vi "_FPGA Set LCD Msg.vi"(4 "Info":string, 5 "ErrNum":string, 6 "error in":errorcluster, 7 "Line2Msg (same)":T1 items=["Same", "Empty", "VacFail", "Cancel", "CheckGas", "EleFail", "Probe1Fail", "Probe2Fail", "HeaterFail", "DoorOpen", "CheckComm", "PressStart", "CheckSource", "VacWarn", "ForelineHigh", "SourceExhaustLow"], 8 "Line1Msg (same)":T2 items=["Same", "Empty", "Connected", "Starting", "Stopping", "Action", "On", "Service", "Call", "Acquiring", "Source"]) -> (0 "error out":errorcluster)   [LabVIEW 2015]
uses:
  Type/_LCD Line1 Msg.ctl
  Type/_LCD Line2 Msg.ctl
  Type/_RT LED Num.ctl
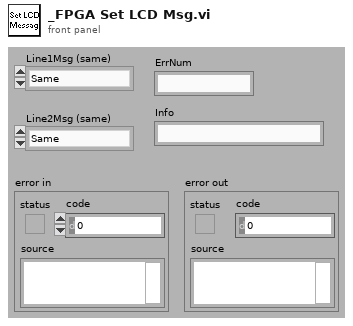
[diagram p1: front panel]
types:
  T1 = typedef "_LCD Line2 Msg.ctl" = u16
  T2 = typedef "_LCD Line1 Msg.ctl" = u16
  T3 = typedef "_RT LED Num.ctl" = enum8{"ReadKey", "ClearKeyBuffer", "ClearLCD", "BacklightOn"}
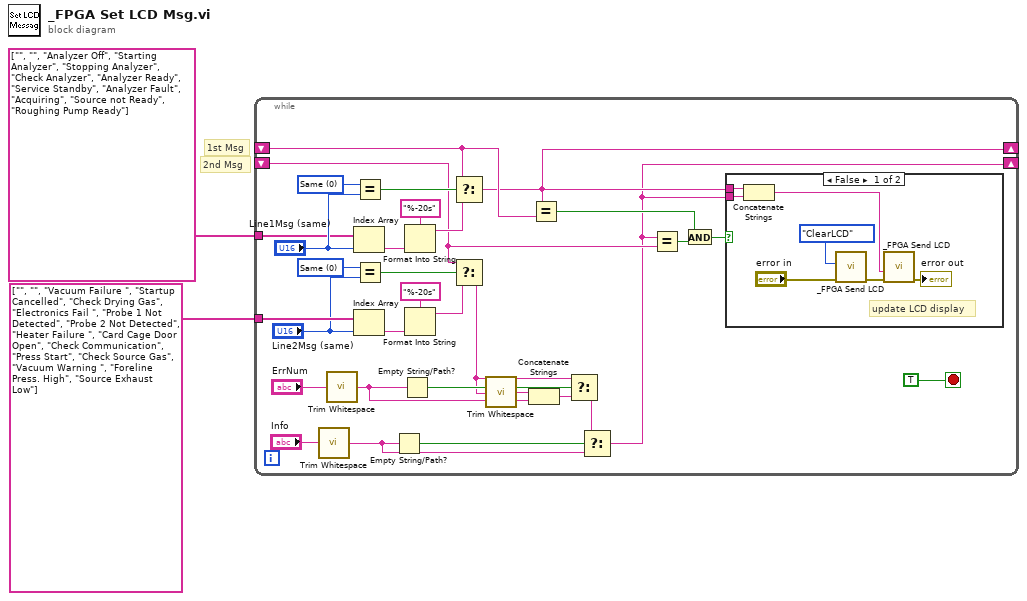
[diagram p0: block diagram]
diagram:
  # "2nd Msg"
  # "1st Msg"
  n1 = while {
    shift-right: [w5] -> _
    shift-left: _ -> [w10]
    shift-right: [w4] -> _
    shift-left: _ -> [w9]
    tunnel: string[] ["", "", "Analyzer Off", "Starting Analyzer", "Stopping Analyzer", "Check Analyzer", "Analyzer Ready", "Service Standby", "Analyzer Fault", "Acquiring", "Source not Ready", "Roughing Pump Ready"] -> [w27]
    tunnel: string[] ["", "", "Vacuum Failure ", "Startup Cancelled", "Check Drying Gas", "Electronics Fail ", "Probe 1 Not Detected", "Probe 2 Not Detected", "Heater Failure ", "Card Cage Door Open", "Check Communication", "Press Start", "Check Source Gas", "Vacuum Warning ", "Foreline Press. High", "Source Exhaust Low"] -> [w22]
    stop <- TRUE stop-if-true
    w20 = T1 0 items=["Same", "Empty", "VacFail", "Cancel", "CheckGas", "EleFail", "Probe1Fail", "Probe2Fail", "HeaterFail", "DoorOpen", "CheckComm", "PressStart", "CheckSource"] ("x")
    w30 = T2 0 items=["Same", "Empty", "Connected", "Starting", "Stopping", "Action", "On", "Service", "Call", "Acquiring", "Source"] ("x")
    n2 = call <vilib>:"Trim Whitespace.vi"("string"="Info") -> ("trimmed string"=w11:string)  [unwired: 1 in]
    n3 = call <vilib>:"Trim Whitespace.vi"("string"="ErrNum") -> ("trimmed string"=w15:string)  [unwired: 1 in]
    n4 = Index Array(array=w27, index="Line1Msg (same)") -> (element=w32:string)
    n5 = Index Array(array=w22, index="Line2Msg (same)") -> (element=w24:string)
    n6 = Equal?(x=w30, y="Line1Msg (same)") -> (x = y?=w29:bool)
    n7 = Equal?(x=w20, y="Line2Msg (same)") -> (x = y?=w25:bool)
    n8 = Empty String/Path?(string/path=w11) -> (empty?=w13:bool)
    n9 = Empty String/Path?(string/path=w15) -> (empty?=w18:bool)
    n10 = Format Into String(format string="%-20s", w32) -> (resulting string=w28:string)  [unwired: 2 in, 1 out]
    n11 = Format Into String(format string="%-20s", w24) -> (resulting string=w26:string)  [unwired: 2 in, 1 out]
    n12 = Select(t=w10, s=w29, f=w28) -> (s? t:f=w5:string)
    n13 = Select(t=w9, s=w25, f=w26) -> (s? t:f=w16:string)
    n14 = call <vilib>:"Trim Whitespace.vi"("string"=w16) -> ("trimmed string"=w3:string)  [unwired: 1 in]
    n15 = Concatenate Strings(w3, w15) -> (w17:string)
    n16 = Equal?(x=w5, y=w10) -> (x = y?=w7:bool)
    n17 = Select(t=w16, s=w18, f=w17) -> (s? t:f=w12:string)
    n18 = Select(t=w12, s=w13, f=w11) -> (s? t:f=w4:string)
    n19 = Equal?(x=w4, y=w9) -> (x = y?=w8:bool)
    n20 = And(x=w7, y=w8) -> (x .and. y?=w6:bool)
    n21 = case shown="False" w6 {
      tunnel: w5 -> [w37 _]
      tunnel: w4 -> [w36 _]
      frame False {
        # "update LCD display"
        n22 = Concatenate Strings(w37, w36) -> (w35:string)
        n23 = call "_FPGA Send LCD.vi"("error in (no error)"="error in", "Command"=_RT_LED_Num."ClearLCD" ("LED#")) -> ("error out"=w39:errorcluster)  [unwired: 3 in, 3 out]
        n24 = call "_FPGA Send LCD.vi"("error in (no error)"=w39, "Message"=w35) -> ("error out"=→"error out":errorcluster)  [unwired: 3 in, 3 out]
      }
      frame True {
      }
    }
  }
